vi "Synchronize.vi"(7 "Retries (3)":i32=3, 8 "Error In":errorcluster, 11 "LINX Device Config":T1) -> (0 "Error Out":errorcluster, 3 "LINX Device Config":T1)   [LabVIEW 2011, in "LVH-LINX.lvlib" / "Device.lvlib"]
doc: "Synchronize the LINX device with LabVIEW."
uses:
  Device.lvlib
  Type Defs/LINX Device Config.ctl
  Type Defs/Interface.ctl
  Type Defs/TCP Config.ctl
  Type Defs/Channels.ctl
  Type Defs/Error Type.ctl
  LVH-LINX.lvlib
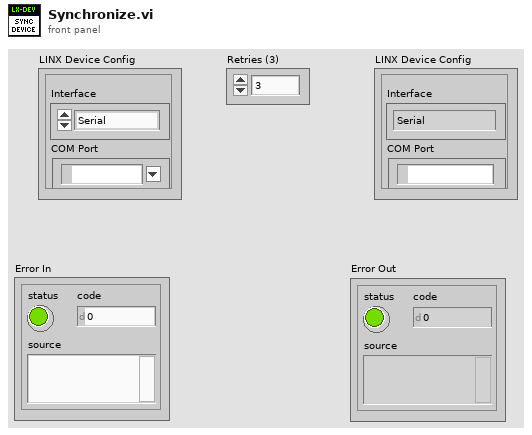
[diagram p1: front panel]
types:
  T1 = typedef "LVH-LINX.lvlib/Device.lvlib/LINX Device Config.ctl" = cluster{"Interface":T2, "COM Port":refnum<visa-resource-name>, "TCP Configuration":T3, "Device Family":u8, "Device ID":u8, "Device Name":string, "TCP Ref":refnum<k5>, "Channels":T4}
  T2 = typedef "LVH-LINX.lvlib/Interface.ctl" = enum16{"Serial", "TCP"}
  T3 = typedef "LVH-LINX.lvlib/Device.lvlib/TCP Config.ctl" = cluster{"IP Address":string, "Port":u16}
  T4 = typedef "LVH-LINX.lvlib/Channels.ctl" = cluster{"DI":u8[], "DO":u8[], "AI":u8[], "AO":u8[], "PWM":u8[], "QE":u8[], "UART":u8[], "I2C 2":u8[], "SPI":u8[], "CAN":u8[], "Servo":u8[], "AI Ref (V)":dbl, "AO Ref (V)":dbl, "AO Resolution (Bits)":u8}
  T5 = typedef "LVH-LINX.lvlib/Error Type.ctl" = enum16{"Unknown", "Timeout", "Corrupt Return Packet", "Unable To Connect", "Command Not Supported", "Channel DNE", "Invalid COM Config", "Firmware Version Mismatch", "myRIO Support", "CMD Specific Error"}
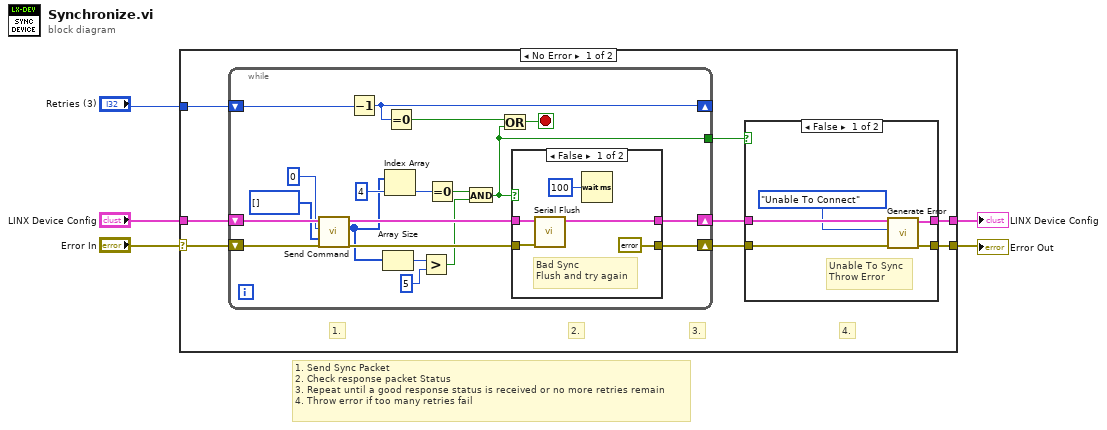
[diagram p0: block diagram]
diagram:
  # "1. Send Sync Packet\n2. Check response packet Status\n3. Repeat until a good response status is received or no more retries remain\n4. Throw error if too many retries fail"
  n1 = case shown="No Error" "Error In" {
    selector: "Error In" -> [w6 w49]
    tunnel: "Retries (3)" -> [w13 _]
    tunnel: "LINX Device Config" -> [w12 w48]
    tunnel: [w8 w48] -> w3
    tunnel: [w7 w49] -> w2
    frame No Error {
      # "4."
      # "3."
      # "2."
      # "1."
      n2 = while {
        shift-right: [w35] -> _
        shift-left: w13 -> [w36]
        shift-right: [w29] -> w10
        shift-left: w6 -> [w39]
        tunnel: [w21] -> w9
        shift-right: [w31] -> w11
        shift-left: w12 -> [w40]
        stop <- w27 stop-if-true
        n3 = call "Send Command.vi"("Error In"=w39, "ARGS"=u8[] [], "CMD"=u16 0, "LINX Device Config"=w40) -> ("Error Out"=w28:errorcluster, "Response"=w26:u8[], "LINX Device Config"=w30:T1)  [unwired: 4 in, 1 out]
        n4 = Decrement(x=w36) -> (x-1=w35:i32)
        n5 = Array Size(array=w26) -> (size(s)=w25:i32)
        n6 = Index Array(array=w26, index=4) -> (element=w33:u8)
        n7 = Equal To 0?(x=w35) -> (x = 0?=w32:bool)
        n8 = Greater?(x=w25, y=5) -> (0:w23:bool)
        n9 = Equal To 0?(x=w33) -> (x = 0?=w22:bool)
        n10 = And(x=w22, y=w23) -> (x .and. y?=w21:bool)
        n11 = Or(x=w32, y=w21) -> (x .or. y?=w27:bool)
        n12 = case shown="False" w21 {
          tunnel: [w42 w47] -> w31
          tunnel: w30 -> [w45 w47]
          tunnel: [errorcluster {"status"=FALSE, "code"=0, "source"=""} ("Error Out") w46] -> w29
          tunnel: w28 -> [w44 w46]
          frame False {
            # "Bad Sync\nFlush and try again"
            n13 = call "Serial Flush.vi"("Error In"=w44, "LINX Device Config"=w45) -> ("LINX Device Config"=w42:T1)  [unwired: 8 in, 1 out]
            n14 = Wait (ms)(milliseconds to wait=u32 100) -> ()  [unwired: 1 out]
          }
          frame True {
            # "Sync OK"
          }
        }
      }
      n15 = case shown="False" w9 {
        tunnel: [w18 w20] -> w8
        tunnel: w11 -> [w16 w20]
        tunnel: [w17 w19] -> w7
        tunnel: w10 -> [w14 w19]
        frame False {
          # "Unable To Sync\nThrow Error"
          n16 = call "Generate Error.vi"("Error In"=w14, "Error Type"=Error_Type."Unable To Connect", "LINX Device Config"=w16) -> ("Error Out"=w17:errorcluster, "LINX Device Config"=w18:T1)  [unwired: 7 in]
        }
        frame True {
          # "Sync OK"
        }
      }
    }
    frame Error {
    }
  }
  "Error Out" <- w2
  "LINX Device Config" <- w3
